vi "TEMPCOUNTER_display.vi"(8 "error out 2":errorcluster, 11 "Enum":enum16{"RESET", "READ", "WRITE"}(ring)) -> (0 "error out":errorcluster, 3 "OUT":dbl)   [LabVIEW 2017]
uses:
  <vilib>/addons/database/Connection.llb/Conn ObjectReference.ctl
  <vilib>/Utility/file.llb/Read Delimited Spreadsheet (DBL).vi
  Globle/Current date.vi
  <vilib>/Utility/file.llb/Write Delimited Spreadsheet (DBL).vi
  <vilib>/addons/database/NI_Database_API.lvlib
panel:
  out "connection reference 2":T1
  in  "connection reference":T1
  out "appended path":path
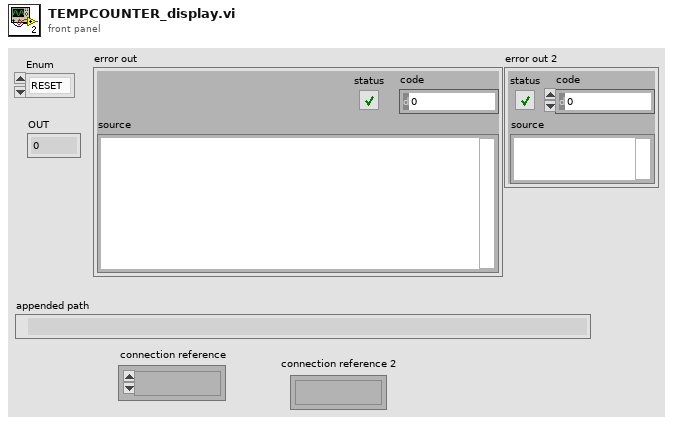
[diagram p1: front panel]
types:
  T1 = typedef "NI_Database_API.lvlib/Conn ObjectReference.ctl" = refnum<k1>
  T2 = enum32{"invalid app kind", "Development System", "Run Time System", "Student Edition", "Embedded LabVIEW", "Evaluation", "Custom"}
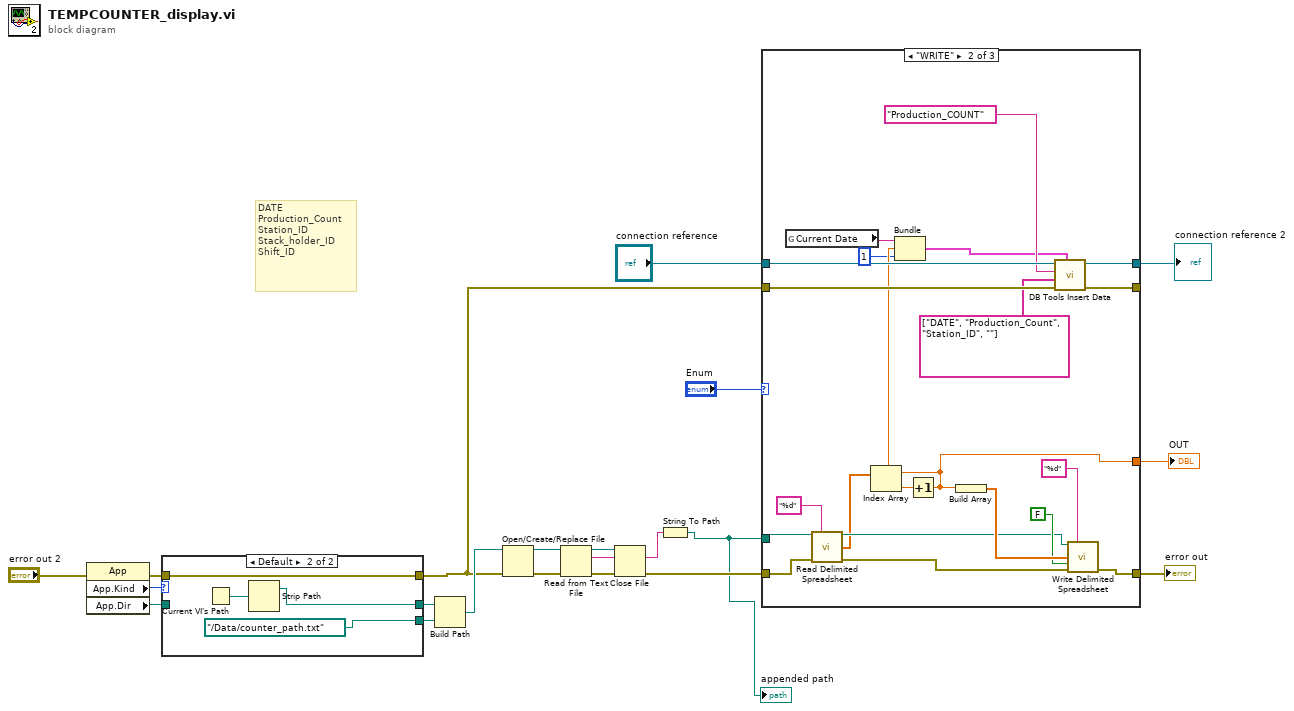
[diagram p0: block diagram]
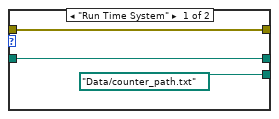
[diagram p2: hidden frame]
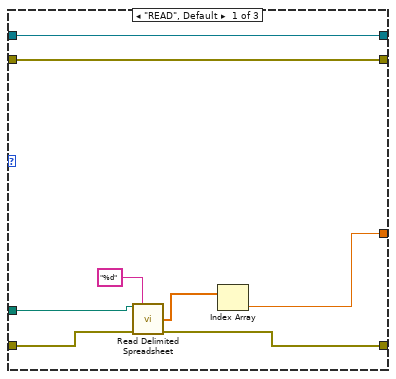
[diagram p3: hidden frame]
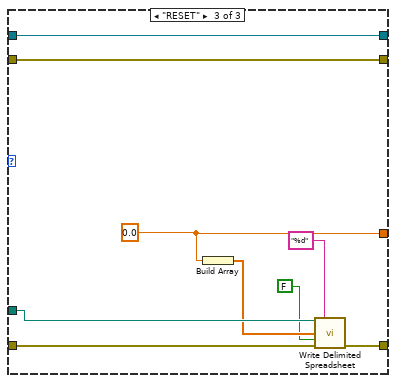
[diagram p4: hidden frame]
diagram:
  # "DATE\nProduction_Count\nStation_ID\nStack_holder_ID\nShift_ID"
  n1 = property class="App"(error in="error out 2") -> (error out=w12:errorcluster, "App.Kind"=w17:T2, "App.Dir"=w16:path)  [unwired: 1 in, 1 out]
  n2 = case shown="Default" w17 {
    tunnel: w16 -> [w23 _]
    tunnel: [path "Data/counter_path.txt" ("path") path "../Data/counter_path.txt" ("path")] -> w15
    tunnel: [w23 w25] -> w14
    tunnel: [w21 w24] -> w2
    tunnel: w12 -> [w21 w24]
    frame "Run Time System" {
    }
    frame Default {
      n3 = Current VI's Path() -> (path=w26:path)
      n4 = Strip Path(path=w26) -> (stripped path=w25:path)  [unwired: 1 out]
    }
  }
  n5 = Build Path(base path=w14, name or relative path=w15) -> (appended path=w5:path)
  n6 = Open/Create/Replace File(file path (use dialog)=w5, error in=w2) -> (refnum out=w11:refnum<file>, error out=w8:errorcluster)  [unwired: 4 in, 1 out]
  n7 = Read from Text File(file (use dialog)=w11, error in=w8) -> (refnum out=w10:refnum<file>, text=w6:string, error out=w9:errorcluster)  [unwired: 2 in, 1 out]
  n8 = Close File(refnum=w10, error in=w9) -> (error out=w7:errorcluster)  [unwired: 1 out]
  n9 = String To Path(string=w6) -> (path=w4:path)
  "appended path" <- w4
  n10 = case shown="\"WRITE\"" "Enum" {
    tunnel: w4 -> [w34 w56 w65]
    tunnel: [w31 w40 w59] -> w19
    tunnel: [w33 w50 w61] -> w18
    tunnel: w7 -> [w30 w46 w60]
    tunnel: "connection reference" -> [w28 w45 w57]
    tunnel: w2 -> [w29 w44 w58]
    tunnel: [w29 w37 w58] -> _
    tunnel: [w28 w36 w57] -> w1
    frame "READ", Default {
      n11 = call-poly <vilib>:"Read Delimited Spreadsheet.vi"("file path (dialog if empty)"=w34, "format (%.3f)"="%d", "error in (no error)"=w30) -> ("first row"=w32:dbl[], "error out"=w33:errorcluster)  [unwired: 7 in, 4 out]
      n12 = Index Array(array=w32) -> (element=w31:dbl)  [unwired: 1 in]
    }
    frame "WRITE" {
      n13 = global read "Current date.vi" "Current Date"() -> (w41:string)
      n14 = call-poly <vilib>:"Read Delimited Spreadsheet.vi"("file path (dialog if empty)"=w56, "format (%.3f)"="%d", "error in (no error)"=w46) -> ("new file path (Not A Path if cancelled)"=w49:path, "first row"=w48:dbl[], "error out"=w51:errorcluster)  [unwired: 7 in, 3 out]
      n15 = Index Array(array=w48) -> (element=w47:dbl)  [unwired: 1 in]
      n16 = Increment(x=w47) -> (x+1=w40:dbl)
      n17 = Bundle("Current Date"=w41, w40, 1) -> (w38:cluster{"Current Date":string, dbl, i32})  [unwired: 1 in]
      n18 = Build Array(w40) -> (w54:dbl[])
      n19 = call <vilib>:"DB Tools Insert Data.vi"("data"=w38, "error in (no error)"=w44, "columns"=string[] ["DATE", "Production_Count", "Station_ID", ""], "table"="Production_COUNT", "connection reference"=w45) -> ("error out"=w37:errorcluster, "connection reference out"=w36:T1)  [unwired: 5 in]
      n20 = call-poly <vilib>:"Write Delimited Spreadsheet.vi"("file path (dialog if empty)"=w49, "format (%.3f)"="%d", "1D data"=w54, "append to file? (new file:F)"=FALSE, "error in (no error)"=w51) -> ("error out"=w50:errorcluster)  [unwired: 9 in, 1 out]
    }
    frame "RESET" {
      w59 = 0.0
      n21 = Build Array(w59) -> (w64:dbl[])
      n22 = call-poly <vilib>:"Write Delimited Spreadsheet.vi"("file path (dialog if empty)"=w65, "format (%.3f)"="%d", "1D data"=w64, "append to file? (new file:F)"=FALSE, "error in (no error)"=w60) -> ("error out"=w61:errorcluster)  [unwired: 9 in, 1 out]
    }
  }
  "OUT" <- w19
  "error out" <- w18
  "connection reference 2" <- w1
